vi "ComputeAstrometry.vi"() -> ()   [LabVIEW 2011]
uses:
  <vilib>/silver_ctls/ArrayMatrixCluster/Real Matrix NI_Silver.ctl
  <vilib>/Analysis/Matrix/Datatypes/RealMatrix.ctl
  <vilib>/Analysis/baseanly.llb/Matrix Type of Inverse Matrix.ctl
  <vilib>/Analysis/baseanly.llb/Real Inverse Matrix.vi
  <vilib>/Analysis/NI_AALBase.lvlib
  <vilib>/Analysis/Matrix/NI_Matrix.lvlib
panel:
  out "error":i32
  out "Inverse Matrix":T1
  out "A":T2
  out "xi":dbl[](array[numeric])
  out "eta":dbl[](array[numeric])
  out "dely2":dbl
  out "dely1":dbl
  out "delx2":dbl
  out "delx1":dbl
  out "Scale (°/pas)":dbl
  in  "Scale (\"/pas)":dbl
  in  "Y":dbl[](array[numeric])
  in  "X":dbl[](array[numeric])
  in  "DEC":dbl[](array[numeric])
  in  "RA":dbl[](array[numeric])
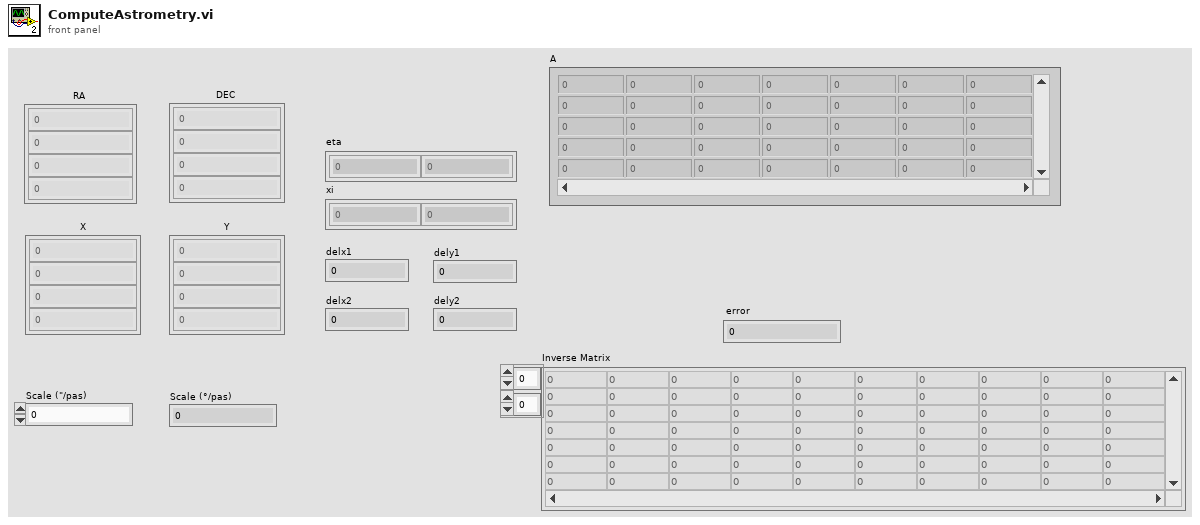
[diagram p1: front panel]
types:
  T1 = typedef "NI_Matrix.lvlib/RealMatrix.ctl" = dbl[][]
  T2 = typedef "Real Matrix NI_Silver.ctl" = dbl[][]
  T3 = cluster{"NAXIS":dbl[], "CD":dbl[][], "CDELT":dbl[], "CRPIX":dbl[], "CTYPE":string[], "CRVAL":dbl[], "LONGPOLE":dbl, "LATPOLE":dbl, "PV2":dbl[]}
  T4 = typedef "NI_AALBase.lvlib/Matrix Type of Inverse Matrix.ctl" = enum32{"General", "Positive Definite", "Lower Triangular", "Upper Triangular"}
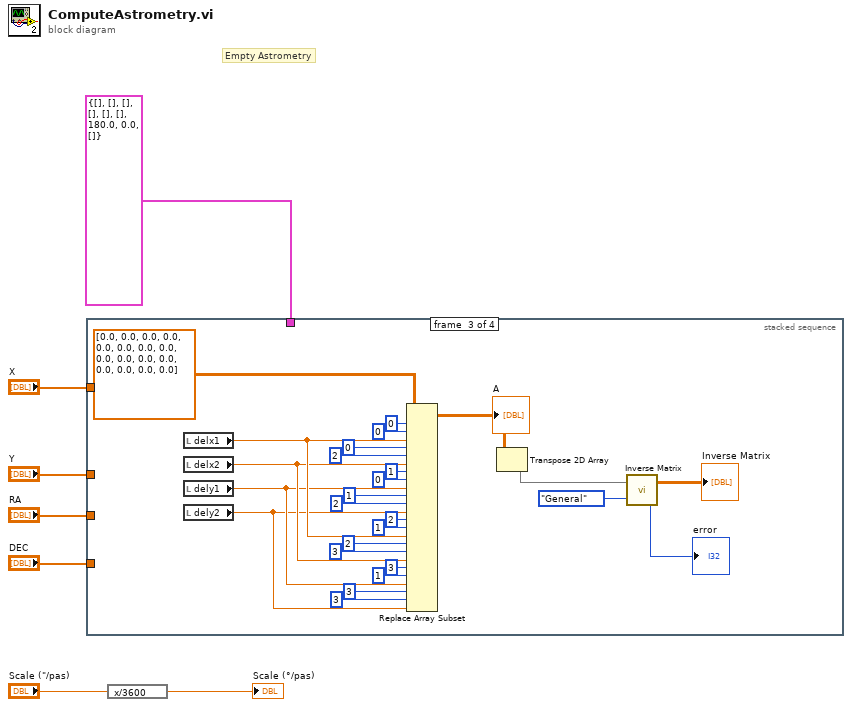
[diagram p0: block diagram]
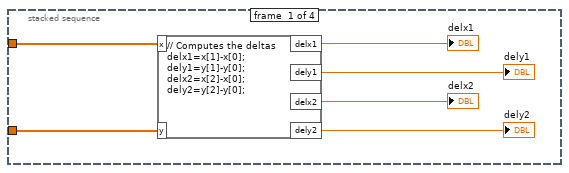
[diagram p2: hidden frame]
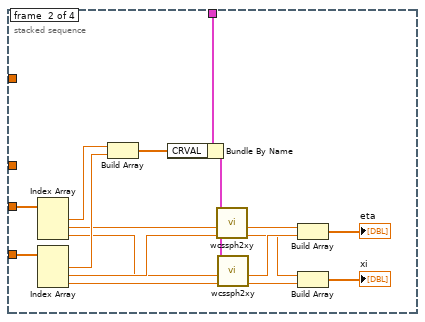
[diagram p3: hidden frame]
diagram:
  # "Empty Astrometry"
  n1 = stacked-sequence {
    tunnel: "X" -> [w9 _ _ _]
    tunnel: "Y" -> [w10 _ _ _]
    tunnel: "RA" -> [_ w28 _ _]
    tunnel: "DEC" -> [_ w27 _ _]
    tunnel: T3 {"NAXIS"=[], "CD"=[], "CDELT"=[], "CRPIX"=[], "CTYPE"=[], "CRVAL"=[], "LONGPOLE"=180.0, "LATPOLE"=0.0, "PV2"=[]} ("Astrometry") -> [_ w25 _ _]
    frame #0 {
      n2 = formula code="// Computes the deltas\ndelx1=x[1]-x[0];\ndely1=y[1]-y[0];\ndelx2=x[2]-x[0];\ndely2=y[2]-y[0];"("x"=w9, "y"=w10) -> ("delx1"=→"delx1":dbl, "dely1"=→"dely1":dbl, "delx2"=→"delx2":dbl, "dely2"=→"dely2":dbl)
    }
    frame #1 {
      n3 = Index Array(array=w28) -> (element #1=w30:dbl, element #2=w24:dbl, element #3=w22:dbl)  [unwired: 3 in]
      n4 = Index Array(array=w27) -> (element #1=w29:dbl, element #2=w23:dbl, element #3=w21:dbl)  [unwired: 3 in]
      n5 = Build Array(w30, w29) -> (w26:dbl[])
      n6 = Bundle By Name(cluster=w25, "CRVAL"=w26) -> (w20:T3)
      n7 = call "wcssph2xy.vi"("lat"=w23, "lon"=w24, "Astrometry"=w20) -> ("Y"=w16:dbl, "X"=w18:dbl)  [unwired: 7 in]
      n8 = call "wcssph2xy.vi"("lat"=w21, "lon"=w22, "Astrometry"=w20) -> ("Y"=w19:dbl, "X"=w17:dbl)  [unwired: 7 in]
      n9 = Build Array(w18, w17) -> (→"eta":dbl[])
      n10 = Build Array(w16, w19) -> (→"xi":dbl[])
    }
    frame #2 {
      n11 = local read "delx1"() -> (w38:dbl)
      n12 = local read "delx2"() -> (w37:dbl)
      n13 = local read "dely1"() -> (w36:dbl)
      n14 = local read "dely2"() -> (w35:dbl)
      n15 = Replace Array Subset(array=T2 [[0.0, 0.0, 0.0, 0.0], [0.0, 0.0, 0.0, 0.0], [0.0, 0.0, 0.0, 0.0], [0.0, 0.0, 0.0, 0.0]] ("A"), new element #1=w38, index (row) #1=0 ("disabled index (row)"), index (col) #1=0 ("disabled index (col)"), new element #2=w37, index (row) #2=0 ("disabled index (row)"), index (col) #2=2 ("disabled index (col)"), new element #3=w36, index (row) #3=1 ("disabled index (row)"), index (col) #3=0 ("disabled index (col)"), new element #4=w35, index (row) #4=1 ("disabled index (row)"), index (col) #4=2 ("disabled index (col)"), new element #5=w38, index (row) #5=2 ("disabled index (row)"), index (col) #5=1 ("disabled index (col)"), new element #6=w37, index (row) #6=2 ("disabled index (row)"), index (col) #6=3 ("disabled index (col)"), new element #7=w36, index (row) #7=3 ("disabled index (row)"), index (col) #7=1 ("disabled index (col)"), new element #8=w35, index (row) #8=3 ("disabled index (row)"), index (col) #8=3 ("disabled index (col)")) -> (w39:T1)
      "A" <- w39
      n16 = Transpose 2D Array(2D array=w39) -> (transposed array=w31:T1)
      n17 = call-poly <vilib>:"Inverse Matrix.vi"("matrix type"=Matrix_Type_of_Inverse_Matrix."General", "Input Matrix"=w31) -> ("error"=→"error":i32, "Inverse Matrix"=→"Inverse Matrix":T1)
    }
    frame #3 {
    }
  }
  n18 = expression code="x/3600"("Scale (\"/pas)") -> (→"Scale (°/pas)":dbl)
